vi "Daq-on-off_1.vi"() -> ()   [LabVIEW 2024]
uses:
  <vilib>/Utility/error.llb/DialogType.ctl
  <vilib>/DAQmx/write.llb/DAQmx Write (Digital Bool 1Line 1Point).vi
  <vilib>/DAQmx/create/channels.llb/DAQmx Create Channel (DO-Digital Output).vi
  <vilib>/DAQmx/miscellaneous.llb/DAQmx Fill In Error Info.vi
panel:
  out "Waveform Chart":i16(graph)
  in  "stop":bool
  out "x-y*floor(x/y)":i32
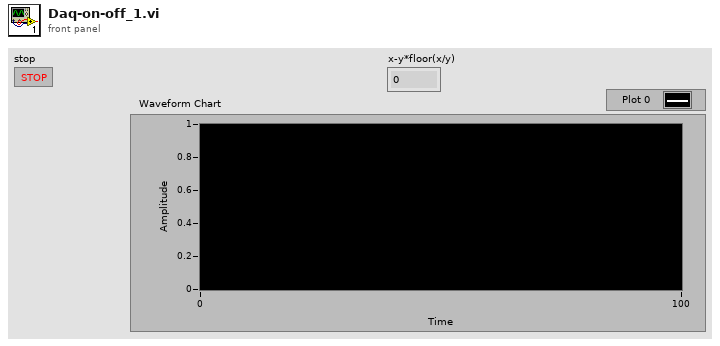
[diagram p1: front panel]
types:
  T1 = typedef "DialogType.ctl" = u16
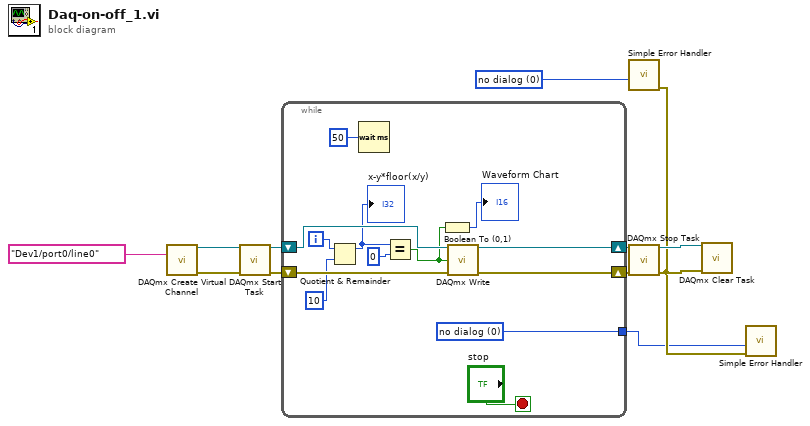
[diagram p0: block diagram]
diagram:
  w2 = T1 0 items=["no dialog", "OK message", "continue or stop message", "OK message + warnings", "continue/stop + warnings"] ("type of dialog (OK msg:1)")
  n1 = call-poly <vilib>:"DAQmx Create Virtual Channel.vi"("lines"=tag "Dev1/port0/line0") -> ("task out"=w11:refnum<k21>, "error out"=w7:errorcluster)  [unwired: 13 in]
  n2 = call <vilib>:"DAQmx Start Task.vi"("task/channels in"=w11, "error in"=w7) -> ("task out"=w10:refnum<k21>, "error out"=w6:errorcluster)  [unwired: 12 in]
  n3 = while {
    tunnel: [w20] -> w3
    shift-right: [w23] -> w9
    shift-left: w10 -> [w24]
    shift-right: [w21] -> w4
    shift-left: w6 -> [w22]
    i -> [w19]
    stop <- "stop" stop-if-true
    w20 = T1 0 items=["no dialog", "OK message", "continue or stop message", "OK message + warnings", "continue/stop + warnings"] ("type of dialog (OK msg:1)")
    n4 = Quotient & Remainder(x=w19, y=10) -> (x-y*floor(x/y)=w14:i32)  [unwired: 1 out]
    "x-y*floor(x/y)" <- w14
    n5 = Wait (ms)(milliseconds to wait=u32 50) -> ()  [unwired: 1 out]
    n6 = Equal?(x=w14, y=0) -> (x = y?=w12:bool)
    n7 = Boolean To (0,1)(Boolean=w12) -> (0, 1=→"Waveform Chart":i16)
    n8 = call-poly <vilib>:"DAQmx Write.vi"("task/channels in"=w24, "data"=w12, "error in"=w22) -> ("task out"=w23:refnum<k21>, "error out"=w21:errorcluster)  [unwired: 10 in, 1 out]
  }
  n9 = call <vilib>:"Simple Error Handler.vi"("type of dialog (OK msg:1)"=w2, "error in (no error)"=w4) -> ()  [unwired: 3 in, 5 out]
  n10 = call <vilib>:"DAQmx Stop Task.vi"("task/channels in"=w9, "error in"=w4) -> ("task out"=w8:refnum<k21>, "error out"=w5:errorcluster)  [unwired: 12 in]
  n11 = call <vilib>:"DAQmx Clear Task.vi"("task in"=w8, "error in"=w5) -> ()  [unwired: 13 in, 1 out]
  n12 = call <vilib>:"Simple Error Handler.vi"("type of dialog (OK msg:1)"=w3, "error in (no error)"=w4) -> ()  [unwired: 3 in, 5 out]
